vi "MotionProfiles_Init.vi"(5 "MP Frame Rate":dbl=5.0 format="%#_13g", 7 "error in (no error)":errorcluster, 8 "CSV File Path":path=path "/home/lvuser/mp.csv", 9 "CAN Talon SRX Ref":T1={"DeviceStatus"={"status"=FALSE, "code"=0, "source"=""}, "Type"=enum."PWM", "PWM"={"PWM Channel"=enum."Invalid", "DeadBand"={"Name"="", "maxPositivePwm"=0, "minPositivePwm"=0, "centerPwm"=0, "maxNegativePwm"=0, "minNegativePwm"=0, "angularRange"=0}}, "CAN"={"Device Number"=0, "SetOutput VI Ref"=variant, "GetOutput VI Ref"=variant, "Enable VI Ref"=variant, "Disable VI Ref"=variant, "Data"=variant}, "Invert"=FALSE}, 10 "MotionProfiles in":refnum<class "MotionProfiles.lvclass">) -> (0 "error out":errorcluster, 3 "MotionProfiles out":refnum<class "MotionProfiles.lvclass">)   [LabVIEW 2016, in "MotionProfiles.lvclass"]
uses:
  MotionProfiles.lvclass
  <vilib>/Rock Robotics/WPI/MotorControl/WPI_MotorControlDeviceRef.ctl
  <vilib>/Rock Robotics/WPI/MotorControl/WPI_MotorControlType.ctl
  <vilib>/Rock Robotics/SystemInterfaces/DIO/FPGA_DIOPWMChannel.ctl
  <vilib>/Rock Robotics/WPI/PWM/WPI_PWMDeadband.ctl
  <vilib>/Rock Robotics/WPI/ThirdParty/CanMotor/TalonSRX/WPI_CANTalonSRX_GlobalOps.ctl
  <vilib>/Rock Robotics/WPI/ThirdParty/CanMotor/TalonSRX/WPI_CANTalonSRX_MotionProfileTrajectoryPt.ctl
  MotionProfile_InternalStateEnum.ctl
  MotionProfile_TalonSetValueEnum.ctl
  MotionProfiles.lvclass/MotionProfiles.ctl
  <vilib>/Utility/file.llb/Read Delimited Spreadsheet (DBL).vi
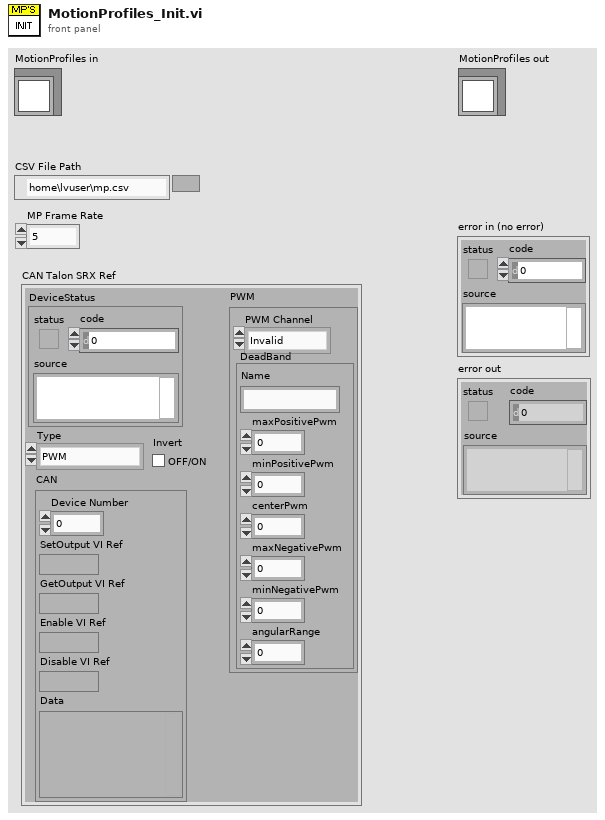
[diagram p1: front panel]
types:
  T1 = typedef "WPI_MotorControlDeviceRef.ctl" = cluster{"DeviceStatus":errorcluster, "Type":T2, "PWM":cluster{"PWM Channel":T3, "DeadBand":T4}, "CAN":cluster{"Device Number":u8, "SetOutput VI Ref":variant, "GetOutput VI Ref":variant, "Enable VI Ref":variant, "Disable VI Ref":variant, "Data":variant}, "Invert":bool}
  T2 = typedef "WPI_MotorControlType.ctl" = enum16{"PWM", "CAN"}
  T3 = typedef "FPGA_DIOPWMChannel.ctl" = enum8{"PWM 0", "PWM 1", "PWM 2", "PWM 3", "PWM 4", "PWM 5", "PWM 6", "PWM 7", "PWM 8", "PWM 9", "PWM MXP 0", "PWM MXP 1", "PWM MXP 2", "PWM MXP 3", "PWM MXP 4", "PWM MXP 5", "PWM MXP 6", "PWM MXP 7", "PWM MXP 8", "PWM MXP 9", "Invalid"}
  T4 = typedef "WPI_PWMDeadband.ctl" = cluster{"Name":string, "maxPositivePwm":i32, "minPositivePwm":i32, "centerPwm":i32, "maxNegativePwm":i32, "minNegativePwm":i32, "angularRange":u16}
  T5 = typedef "MotionProfiles.lvclass/MotionProfile_TalonSetValueEnum.ctl" = enum16{"Disable", "Enable", "Hold"}
  T6 = typedef "MotionProfiles.lvclass/MotionProfile_InternalStateEnum.ctl" = enum16{"Nothing", "Send Points to Talon", "Run Profile"}
  T7 = typedef "WPI_CANTalonSRX_MotionProfileTrajectoryPt.ctl" = cluster{"Duration Ms":u8, "Velocity":dbl, "Position":dbl, "Profile Slot Select":u8, "Is Last":bool, "Velocity Only":bool, "Zero Position":bool, "Compress Code":u8, "Same Velocity":i32, "Delta Position":i32, "Count":u8}
  T8 = typedef "WPI_CANTalonSRX_GlobalOps.ctl" = enum16{"Read For Send", "Write After Receive General", "Write After Receive Feedback", "Write After Receive Encoder", "Write After Receive Ain", "Write Error", "Get All", "Set Output", "Set Mode", "Set Master ID", "Set Brake Mode", "Set Reverse Feedback Sensor", "Set Reverse Closed Loop Output", "Set Override Limits", "Set Forward Limit Enabled", "Set Reverse Limit Enabled", "Set Feedback Select", "Set Profile Select", "Set Throttle Ramp Rate", "Disable", "Set Enc Codes Per Rev", "Set Num Pot Turns", "Set Control Frame Rate", "Enable Legacy Control", "Write After Receive Pulse Width", "Set Enable Frame Rate", "Write After Receive Motion Profile", "Set Motion Profile Flow Control", "Set Motion Profile Control Frame Rate", "Set Current Limit Enable", "Set Usage Frame", "Write After Receive Motion Magic"}
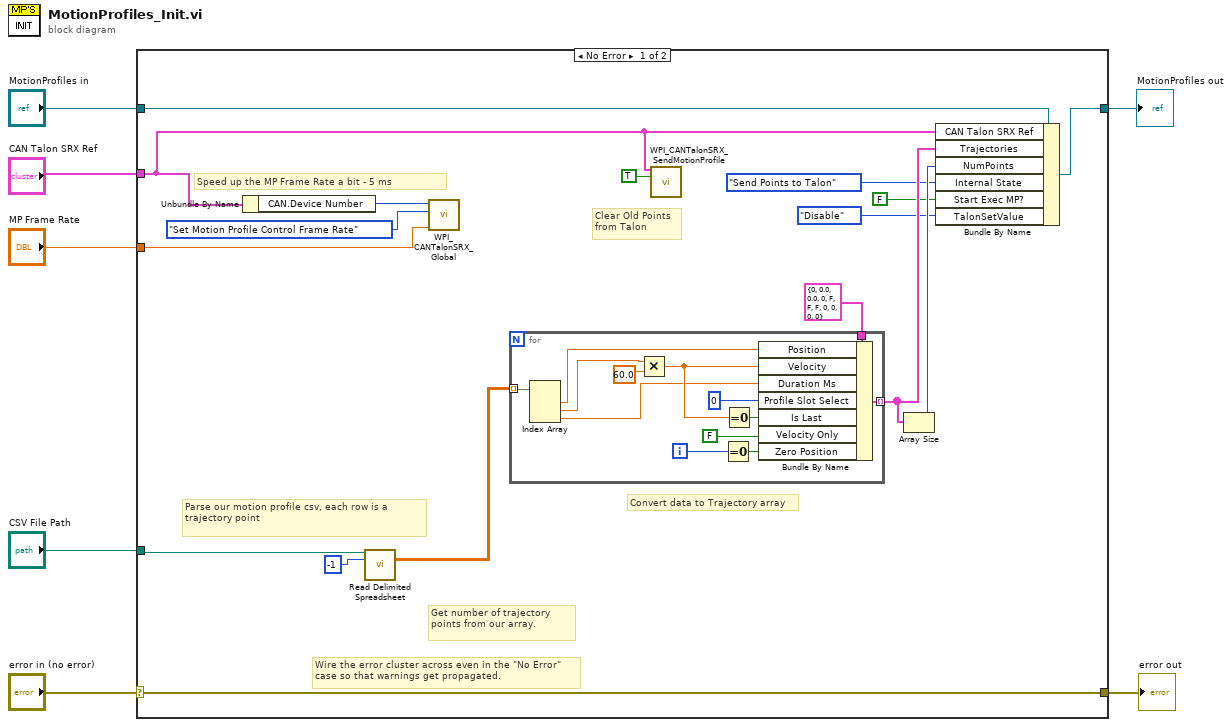
[diagram p0: block diagram]
diagram:
  n1 = case shown="No Error" "error in (no error)" {
    selector: "error in (no error)" -> [w24 w39]
    tunnel: [w24 w39] -> w6
    tunnel: [w22 w38] -> w4
    tunnel: "MotionProfiles in" -> [w23 w38]
    tunnel: "CAN Talon SRX Ref" -> [w8 _]
    tunnel: "CSV File Path" -> [w20 _]
    tunnel: "MP Frame Rate" -> [w17 _]
    frame No Error {
      # "Clear Old Points\nfrom Talon"
      # "Convert data to Trajectory array"
      # "Speed up the MP Frame Rate a bit - 5 ms"
      # "Get number of trajectory points from our array."
      # "Parse our motion profile csv, each row is a trajectory point"
      # "Wire the error cluster across even in the \"No Error\"\ncase so that warnings get propagated."
      n2 = Unbundle By Name(w8) -> ("CAN.Device Number"=w19:u8)
      n3 = call-poly <vilib>:"Read Delimited Spreadsheet.vi"("file path (dialog if empty)"=w20, "number of rows (all:-1)"=-1) -> ("all rows"=w16:dbl[][])  [unwired: 8 in, 5 out]
      n4 = call <vilib>:"WPI_CANTalonSRX_Global.vi"("Set Number"=w17, "Operation"=WPI_CANTalonSRX_GlobalOps."Set Motion Profile Control Frame Rate", "Device ID (0)"=w19) -> ()  [unwired: 6 in, 3 out]
      n5 = for {
        tunnel: [w34] -> w14 mode=indexing
        tunnel: w16 -> [w29] mode=indexing
        tunnel: T7 {"Duration Ms"=0, "Velocity"=0.0, "Position"=0.0, "Profile Slot Select"=0, "Is Last"=FALSE, "Velocity Only"=FALSE, "Zero Position"=FALSE, "Compress Code"=0, "Same Velocity"=0, "Delta Position"=0, "Count"=0} -> [w28]
        i -> [w33]
        n6 = Index Array(array=w29) -> (element #1=w27:dbl, element #2=w26:dbl, element #3=w25:dbl)  [unwired: 3 in]
        n7 = Multiply(x=w26, y=60.0) -> (x*y=w31:dbl)
        n8 = Equal To 0?(x=w33) -> (x = 0?=w35:bool)
        n9 = Equal To 0?(x=w31) -> (x = 0?=w36:bool)
        n10 = Bundle By Name(cluster=w28, "Position"=w27, "Velocity"=w31, "Duration Ms"=w25, "Profile Slot Select"=u8 0, "Is Last"=w36, "Velocity Only"=FALSE, "Zero Position"=w35) -> (w34:T7)
      }
      n11 = call <vilib>:"WPI_CANTalonSRX_SendMotionProfile.vi"("CAN Talon SRX Ref"=w8, "Clear"=TRUE) -> ()  [unwired: 10 in, 4 out]
      n12 = Array Size(array=w14) -> (size(s)=w13:i32)
      n13 = Bundle By Name(cluster=w23, "CAN Talon SRX Ref"=w8, "Trajectories"=w14, "NumPoints"=w13, "Internal State"=MotionProfile_InternalStateEnum."Send Points to Talon", "Start Exec MP?"=FALSE, "TalonSetValue"=MotionProfile_TalonSetValueEnum."Disable") -> (w22:refnum<class "MotionProfiles.lvclass">)
    }
    frame Error {
    }
  }
  "error out" <- w6
  "MotionProfiles out" <- w4
